vi "Configure Log Plot.vi"(0 "VISA resource name":refnum<visa-resource-name>, 1 "Log Plot Measurement Type (1: Signal Phase Noise)":i32(ring)=1 items=["Average Noise Level Floor", "Signal Phase Noise"], 2 "Video Resolution Bandwidth Ratio (1)":dbl=1.0, 3 "Average Count (0)":dbl, 4 "Y-Axis Reference Level (0 dBc/Hz)":dbl, 5 "error in (no error)":errorcluster, 6 "Auto Span to Resolution Bandwidth Ratio (T: Enable)":bool=TRUE, 7 "Start Offset (100 Hz)":dbl=100.0 format="%^#_6g", 8 "Manual Span to Resolution Bandwidth Ratio (10)":dbl=10.0, 9 "Stop Offset (1 MHz)":dbl=1000000.0 format="%^#_6g", 11 "Enable DANL Cancellation (Disable)":bool) -> (14 "VISA resource name out":refnum<visa-resource-name>, 19 "error out":errorcluster)   [LabVIEW 2014, in "Agilent ESA PSA Series.lvlib"]
doc: "Configures the Log Plot measurement options of the Phase Noise personality.\n\n<B>Note:</B>\n\nThis VI is only valid in Phase Noise personality. Use <B>Switch Personality</B> VI to switch to Phase Noise before calling this VI."
uses:
  Agilent ESA PSA Series.lvlib
panel:
  # "Only valid for PSA Models"
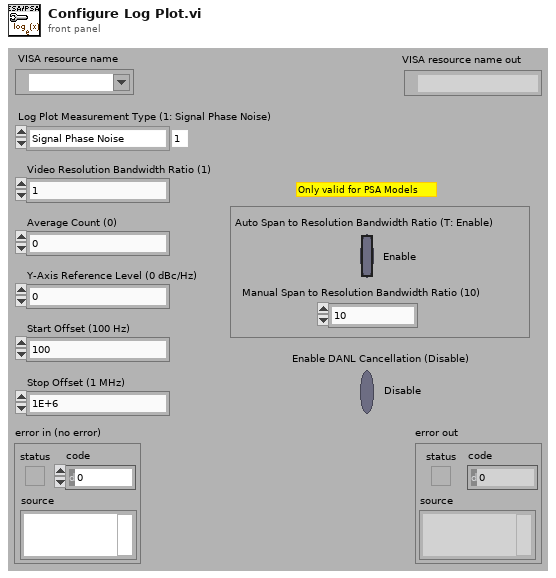
[diagram p1: front panel]
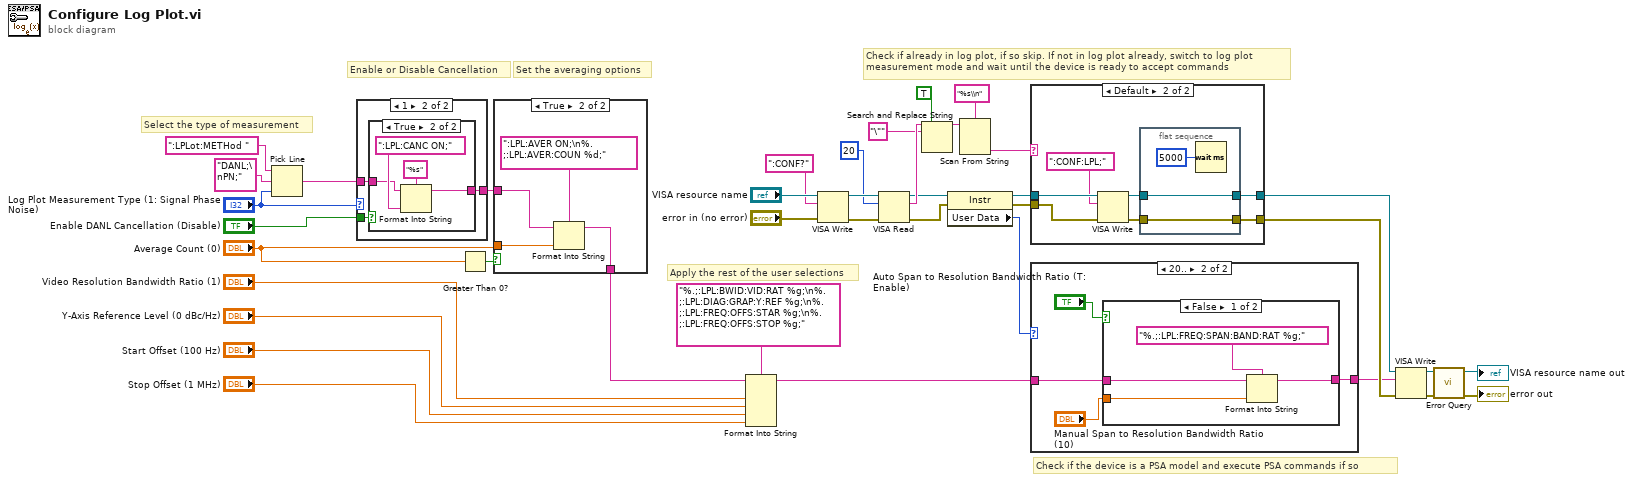
[diagram p0: block diagram]
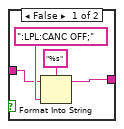
[diagram p3: hidden frame]
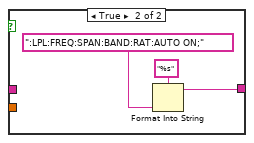
[diagram p6: hidden frame]
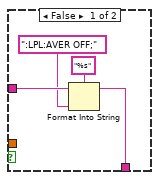
[diagram p7: hidden frame]
diagram:
  # "Enable or Disable Cancellation"
  # "Apply the rest of the user selections"
  # "Set the averaging options"
  # "Select the type of measurement"
  # "Check if already in log plot, if so skip. If not in log plot already, switch to log plot\nmeasurement mode and wait until the device is ready to accept commands"
  # "Check if the device is a PSA model and execute PSA commands if so"
  n1 = Pick Line(string ("")=":LPLot:METHod ", multi-line string="DANL;\nPN;", line index="Log Plot Measurement Type (1: Signal Phase Noise)") -> (output string=w6:string)
  n2 = case shown="1" "Log Plot Measurement Type (1: Signal Phase Noise)" {
    tunnel: "Enable DANL Cancellation (Disable)" -> [_ w43]
    tunnel: w6 -> [w40 w42]
    tunnel: [w40 w41] -> w5
    frame 0, Default {
      # "Measuring noise\nfloor, cancellation\nis cancelled\nautomatically."
    }
    frame 1 {
      n3 = case shown="True" w43 {
        tunnel: [w45 w49] -> w41
        tunnel: w42 -> [w44 w48]
        frame False {
          n4 = Format Into String(format string="%s", initial string=w44, ":LPL:CANC OFF;" ("format string")) -> (resulting string=w45:string)  [unwired: 1 in, 1 out]
        }
        frame True {
          n5 = Format Into String(format string="%s", initial string=w48, ":LPL:CANC ON;" ("format string")) -> (resulting string=w49:string)  [unwired: 1 in, 1 out]
        }
      }
    }
  }
  n6 = Greater Than 0?(x="Average Count (0)") -> (x > 0?=w36:bool)
  n7 = case shown="True" w36 {
    tunnel: "Average Count (0)" -> [_ w59]
    tunnel: w5 -> [w55 w57]
    tunnel: [w54 w56] -> w34
    frame False {
      n8 = Format Into String(format string="%s", initial string=w55, ":LPL:AVER OFF;" ("input 1")) -> (resulting string=w54:string)  [unwired: 1 in, 1 out]
    }
    frame True {
      n9 = Format Into String(format string=":LPL:AVER ON;\n%.;:LPL:AVER:COUN %d;", initial string=w57, w59) -> (resulting string=w56:string)  [unwired: 1 in, 1 out]
    }
  }
  n10 = Format Into String(format string="%.;:LPL:BWID:VID:RAT %g;\n%.;:LPL:DIAG:GRAP:Y:REF %g;\n%.;:LPL:FREQ:OFFS:STAR %g;\n%.;:LPL:FREQ:OFFS:STOP %g;", initial string=w34, "Video Resolution Bandwidth Ratio (1)", "Y-Axis Reference Level (0 dBc/Hz)", "Start Offset (100 Hz)", "Stop Offset (1 MHz)") -> (resulting string=w1:string)  [unwired: 1 in, 1 out]
  n11 = VISA Write(VISA resource name="VISA resource name", write buffer=":CONF?", error in (no error)="error in (no error)") -> (VISA resource name out=w14:refnum<visa-resource-name>, error out=w13:errorcluster)  [unwired: 1 out]
  n12 = VISA Read(VISA resource name=w14, byte count=u32 20, error in (no error)=w13) -> (VISA resource name out=w10:refnum<visa-resource-name>, read buffer=w19:string, error out=w9:errorcluster)  [unwired: 1 out]
  n13 = Search and Replace String(replace all?=TRUE ("replace all? (F)"), input string=w19, search string="\"") -> (result string=w16:string)  [unwired: 5 in, 3 out]
  n14 = property class="Instr"(reference=w10, error in=w9) -> (reference out=w30:refnum<visa-resource-name>, error out=w29:errorcluster, "User Data"=w31:u32)
  n15 = Scan From String(format string="%s\\n", input string=w16) -> (output 1=w11:string)  [unwired: 3 in, 3 out]
  n16 = case shown="Default" w11 {
    tunnel: w30 -> [w61 w68]
    tunnel: w29 -> [w60 w67]
    tunnel: [w61 w64] -> w28
    tunnel: [w60 w63] -> w27
    frame "LPL", "LPLot" {
    }
    frame Default {
      n17 = VISA Write(VISA resource name=w68, write buffer=":CONF:LPL;", error in (no error)=w67) -> (VISA resource name out=w66:refnum<visa-resource-name>, error out=w65:errorcluster)  [unwired: 1 out]
      n18 = flat-sequence {
        tunnel: w66 -> [w71]
        tunnel: w65 -> [w70]
        tunnel: [w71] -> w64
        tunnel: [w70] -> w63
        frame #0 {
          n19 = Wait (ms)(milliseconds to wait=u32 5000) -> ()  [unwired: 1 out]
        }
      }
    }
  }
  n20 = case shown="20.." w31 {
    tunnel: [w72 w74] -> w23
    tunnel: w1 -> [w72 w73]
    frame 0..19, Default {
      # "Not a PSA model, therefore skip PSA commands"
    }
    frame 20.. {
      n21 = case shown="False" "Auto Span to Resolution Bandwidth Ratio (T: Enable)" {
        tunnel: [w80 w81] -> w74
        tunnel: "Manual Span to Resolution Bandwidth Ratio (10)" -> [w79 _]
        tunnel: w73 -> [w77 _]
        frame False {
          n22 = Format Into String(format string="%.;:LPL:FREQ:SPAN:BAND:RAT %g;", initial string=w77, w79) -> (resulting string=w80:string)  [unwired: 1 in, 1 out]
        }
        frame True {
          n23 = Format Into String(format string="%s", ":LPL:FREQ:SPAN:BAND:RAT:AUTO ON;") -> (resulting string=w81:string)  [unwired: 2 in, 1 out]
        }
      }
    }
  }
  n24 = VISA Write(VISA resource name=w28, write buffer=w23, error in (no error)=w27) -> (VISA resource name out=w26:refnum<visa-resource-name>, error out=w25:errorcluster)  [unwired: 1 out]
  n25 = call "Error Query.vi"("error in (no error)"=w25, "VISA resource name"=w26) -> ("error out"=→"error out":errorcluster, "VISA resource name out"=→"VISA resource name out":refnum<visa-resource-name>)  [unwired: 6 in, 2 out]
